vi "GraphLine.vi"(0 "xp":dbl, 5 "yp":dbl, 7 "alpha":dbl, 9 "xmax":u32, 11 "ymax":u32) -> (6 "Start Point":cluster{"X":i32, "Y":i32}, 10 "End Point":cluster{"X":i32, "Y":i32})   [LabVIEW 2015]
panel:
  in  "xmin":u32
  in  "ymin":u32
  out "b":dbl
  out "m":dbl
  out "y1":dbl
  out "x1":dbl
  out "y0":dbl
  out "x0":dbl
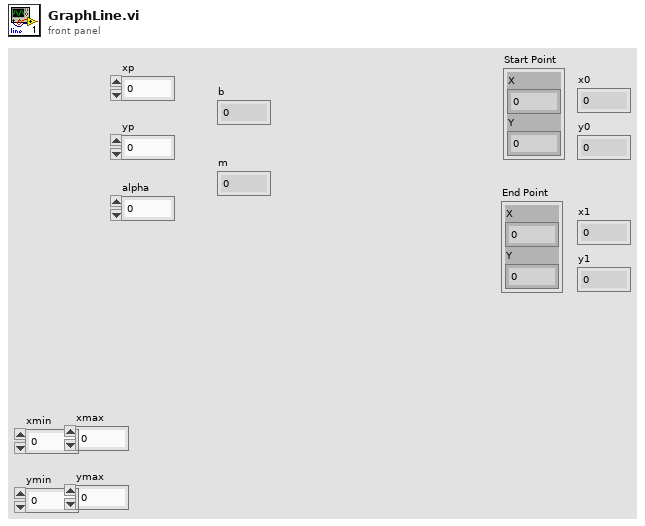
[diagram p1: front panel]
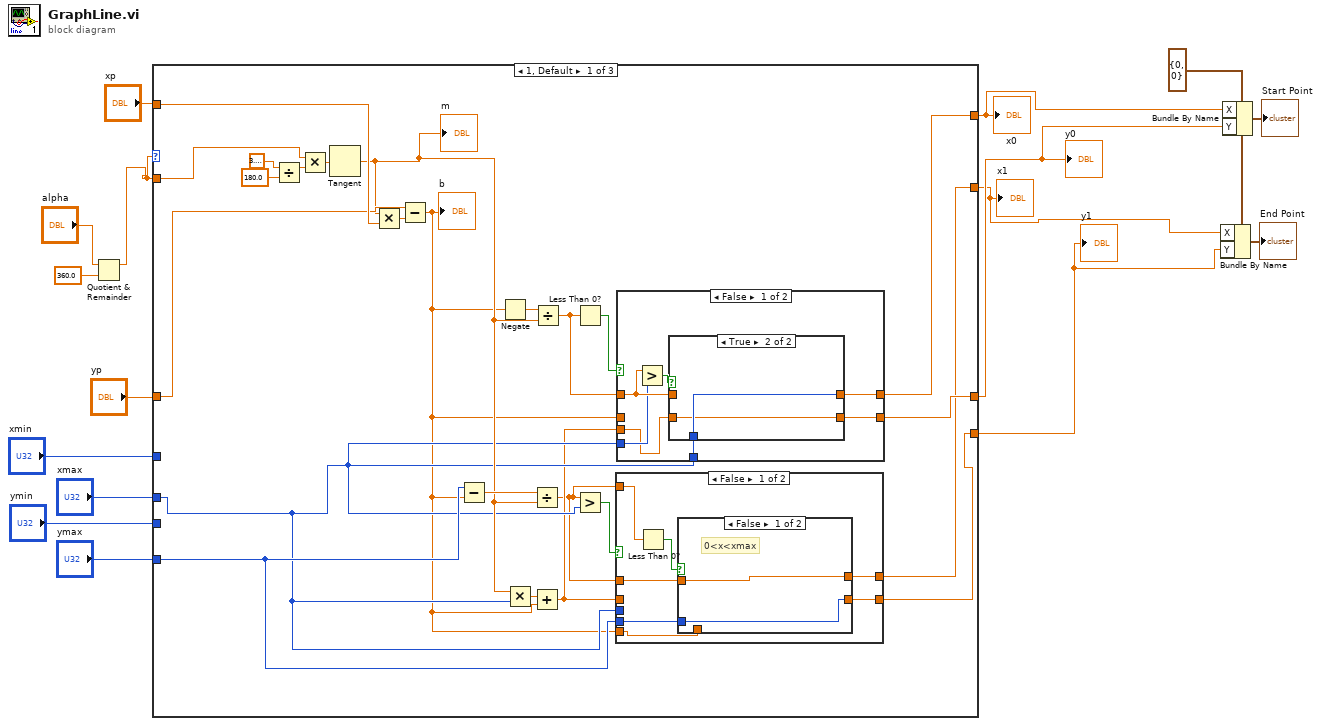
[diagram p0: block diagram]
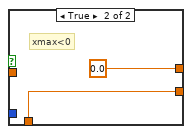
[diagram p2: hidden frame]
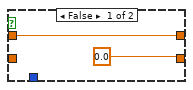
[diagram p4: hidden frame]
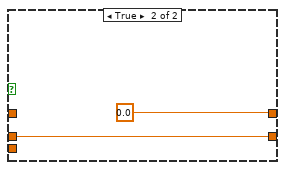
[diagram p5: hidden frame]
diagram:
  w7 = cluster{"X":i32, "Y":i32} {"X"=0, "Y"=0} ("Start Point")
  n1 = Quotient & Remainder(x="alpha", y=360.0) -> (x-y*floor(x/y)=w8:dbl)  [unwired: 1 out]
  n2 = case shown="1, Default" w8 {
    tunnel: w8 -> [w36 _ _]
    tunnel: "yp" -> [w33 _ w72]
    tunnel: "xp" -> [w34 w67 _]
    tunnel: [w28 w69 w72] -> w5
    tunnel: [w22 w68 w72] -> w3
    tunnel: [w30 w67 w71] -> w6
    tunnel: "xmin" -> [_ _ w71]
    tunnel: [w23 w67 w70] -> w4
    tunnel: "xmax" -> [w20 _ w70]
    tunnel: "ymin" -> [_ w69 _]
    tunnel: "ymax" -> [w21 w68 _]
    frame 1, Default {
      n3 = Divide(x=3.141592653589793, y=180.0) -> (x/y=w39:dbl)
      n4 = Multiply(x=w36, y=w39) -> (x*y=w40:dbl)
      n5 = Tangent(1:w40) -> (0:w25:dbl)
      "m" <- w25
      n6 = Multiply(x=w25, y=w34) -> (x*y=w35:dbl)
      n7 = Subtract(x=w33, y=w35) -> (x-y=w17:dbl)
      "b" <- w17
      n8 = Subtract(x=w21, y=w17) -> (x-y=w27:dbl)
      n9 = Negate(x=w17) -> (-x=w32:dbl)
      n10 = Multiply(x=w25, y=w20) -> (x*y=w26:dbl)
      n11 = Divide(x=w27, y=w25) -> (x/y=w18:dbl)
      n12 = Add(x=w26, y=w17) -> (x+y=w19:dbl)
      n13 = Divide(x=w32, y=w25) -> (x/y=w29:dbl)
      n14 = Less Than 0?(x=w29) -> (x < 0?=w31:bool)
      n15 = Greater?(x=w18, y=w20) -> (0:w24:bool)
      n16 = case shown="False" w24 {
        tunnel: [w46 w52] -> w23
        tunnel: w18 -> [w45 _]
        tunnel: [w44 w53] -> w22
        tunnel: w19 -> [_ w53]
        tunnel: w20 -> [_ w52]
        tunnel: w21 -> [w43 _]
        tunnel: w18 -> [w47 _]
        tunnel: w17 -> [w41 _]
        frame False {
          n17 = Less Than 0?(x=w47) -> (x < 0?=w42:bool)
          n18 = case shown="False" w42 {
            tunnel: [w49 0.0] -> w46
            tunnel: w45 -> [w49 _]
            tunnel: [w48 w50] -> w44
            tunnel: w43 -> [w48 _]
            tunnel: w41 -> [_ w50]
            frame False {
              # "0<x<xmax"
            }
            frame True {
              # "xmax<0"
            }
          }
        }
        frame True {
        }
      }
      n19 = case shown="False" w31 {
        tunnel: [w59 0.0] -> w30
        tunnel: w29 -> [w58 _]
        tunnel: [w60 w65] -> w28
        tunnel: w17 -> [_ w65]
        tunnel: w20 -> [w57 _]
        tunnel: w20 -> [w55 _]
        tunnel: w19 -> [w54 _]
        frame False {
          n20 = Greater?(x=w58, y=w57) -> (0:w56:bool)
          n21 = case shown="True" w56 {
            tunnel: [0.0 ("y") w63] -> w60
            tunnel: [w62 w64] -> w59
            tunnel: w58 -> [w62 _]
            tunnel: w55 -> [_ w64]
            tunnel: w54 -> [_ w63]
            frame False {
            }
            frame True {
            }
          }
        }
        frame True {
        }
      }
    }
    frame 90, 270 {
    }
    frame 0 {
    }
  }
  "x0" <- w6
  "y0" <- w5
  "x1" <- w4
  "y1" <- w3
  n22 = Bundle By Name(cluster=w7, "X"=w4, "Y"=w3) -> (→"End Point":cluster{"X":i32, "Y":i32})
  n23 = Bundle By Name(cluster=w7, "X"=w6, "Y"=w5) -> (→"Start Point":cluster{"X":i32, "Y":i32})
